vi "Populate All Fields.vi"(8 "error in (no error)":errorcluster, 11 "Panel Form Controller in":refnum<class "Panel Form Controller.lvclass">) -> (0 "error out":errorcluster, 3 "Panel Form Controller out":refnum<class "Panel Form Controller.lvclass">)   [LabVIEW 2020, in "Panel Form Controller.lvlib" / "Panel Form Controller.lvclass"]
uses:
  Panel Form Controller.lvclass
  Panel Form Controller.lvclass/Panel Form Controller.ctl
  source/Field/Field.lvclass
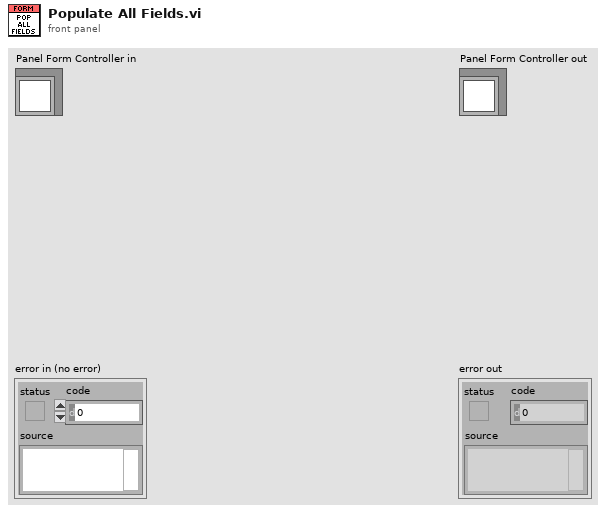
[diagram p1: front panel]
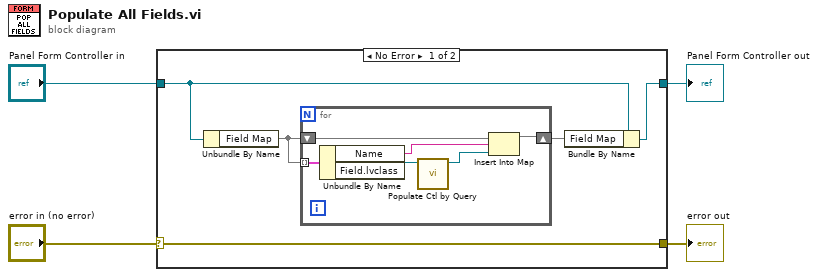
[diagram p0: block diagram]
diagram:
  n1 = case shown="No Error" "error in (no error)" {
    selector: "error in (no error)" -> [w9 w17]
    tunnel: [w9 w17] -> w3
    tunnel: [w5 w16] -> w1
    tunnel: "Panel Form Controller in" -> [w6 w16]
    frame No Error {
      n2 = Unbundle By Name(w6) -> ("Field Map"=w8:map{string, refnum<class "Field.lvclass">})
      n3 = for {
        tunnel: w8 -> [w14] mode=indexing
        shift-right: [w12] -> w7
        shift-left: w8 -> [w13]
        n4 = Unbundle By Name(w14) -> ("Name"=w11:string, "Field.lvclass"=w15:refnum<class "Field.lvclass">)
        n5 = call-dynamic "Populate Ctl by Query.vi"("Field in"=w15) -> ("Field out"=w10:refnum<class "Field.lvclass">)  [unwired: 9 in, 1 out]
        n6 = Insert Into Map(map in=w13, key=w11, value=w10) -> (map out=w12:map{string, refnum<class "Field.lvclass">})  [unwired: 2 out]
      }
      n7 = Bundle By Name(cluster=w6, "Field Map"=w7) -> (w5:refnum<class "Panel Form Controller.lvclass">)
    }
    frame Error {
    }
  }
  "error out" <- w3
  "Panel Form Controller out" <- w1
